vi "Initialize FGEN.vi"(8 "error in (no error)":errorcluster, 10 "FGEN Settings":T2, 11 "measurement context in":refnum<class "Measure Call Context.lvclass">) -> (0 "error out":errorcluster, 1 "Total Wfm Duration (s)":dbl, 2 "FGEN Sessions":T1, 3 "measurement context out":refnum<class "Measure Call Context.lvclass">)   [LabVIEW 2025, in "FGEN Arb Sequence Mode.lvclass"]
uses:
  FGEN Arb Sequence Mode.lvclass
  <vilib>/Plug-In SDKs/Measurements/Measure Call Context/Measure Call Context.lvclass
  <vilib>/Plug-In SDKs/Clients/Session Management V1/Session Reservation/Session Reservation.lvclass
  <instrlib>/niFgen/niFgen.llb/niFgen Output Mode.ctl
  <instrlib>/niFgen/niFgen.llb/niFgen Trigger Mode.ctl
  <vilib>/Plug-In SDKs/Clients/Session Management V1/Session Reservation/Initialize and Close Session Behavior.ctl
  <vilib>/Plug-In SDKs/Measurements/Measure Call Context/Reserve Sessions - NPin.vi
  <vilib>/Plug-In SDKs/Sessions/niFGEN/Initialize Sessions - 1Sess.vi
  <instrlib>/niFgen/niFgen.llb/niFgen Disable Start Trigger.vi
  <instrlib>/niFgen/niFgen.llb/niFgen Create Waveform (DBL).vi
  FGEN Arb Sequence Mode.lvclass/FGEN Arb Sequence Mode.ctl
  <vilib>/Plug-In SDKs/Sessions/niFGEN/NI Session Management niFGEN.lvlib
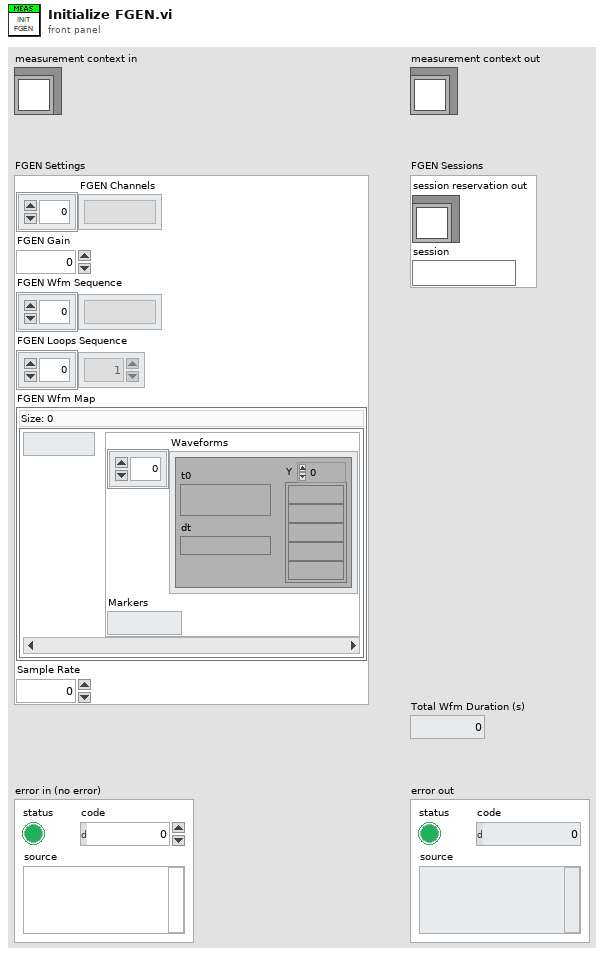
[diagram p1: front panel]
types:
  T1 = cluster{"session reservation out":refnum<class "Session Reservation.lvclass">, "session":refnum<k15>}
  T2 = cluster{"FGEN Channels":string[], "FGEN Gain":dbl, "FGEN Wfm Sequence":string[], "FGEN Loops Sequence":u32[], "FGEN Wfm Map":map{string, cluster{"Waveforms":waveform(dbl)[], "Markers":dbl}}, "Sample Rate":dbl}
  T3 = typedef "NI Session Management V1 Client.lvlib/Session Reservation.lvclass/Initialize and Close Session Behavior.ctl" = enum16{"Auto", "Initialize and Close", "Attach and Detach", "Initialize and Detach", "Attach and Close"}
  T4 = cluster{"Markers":i32, "Waveform Handle":i32, "Wfm Duration":dbl}
  T5 = map{string, cluster{"Markers":i32, "Waveform Handle":i32, "Wfm Duration":dbl}}
  T6 = typedef "niFgen Trigger Mode.ctl" = i32
  T7 = typedef "niFgen Output Mode.ctl" = u32
  T8 = map{string, cluster{"Waveforms":waveform(dbl)[], "Markers":dbl}}
  T9 = cluster{"Waveforms":waveform(dbl)[], "Markers":dbl}
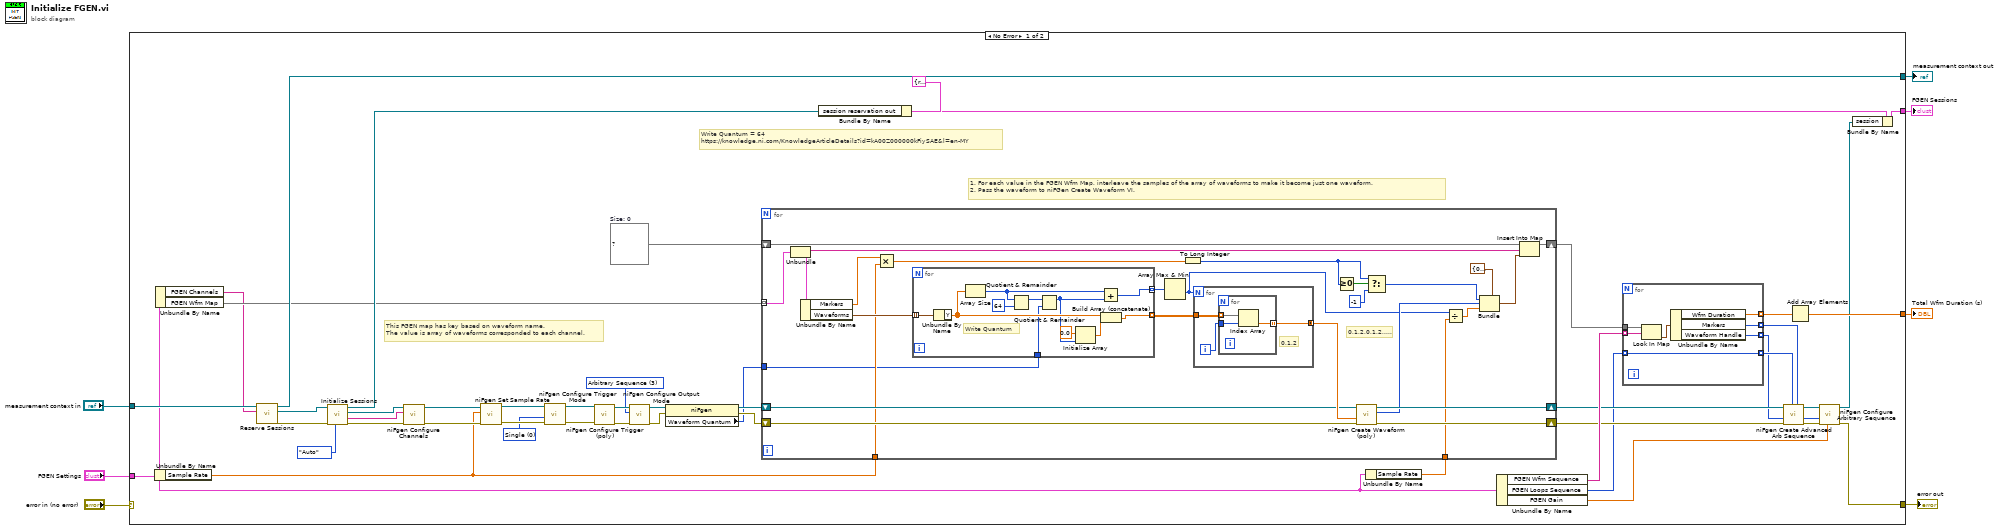
[diagram p0: block diagram]
diagram:
  n1 = case shown="No Error" "error in (no error)" {
    selector: "error in (no error)" -> [_ w109]
    tunnel: [w47 w109] -> w7
    tunnel: "FGEN Settings" -> [w22 _]
    tunnel: [w25 _] -> w4
    tunnel: "measurement context in" -> [w45 w108]
    tunnel: [w20 _] -> w2
    tunnel: [w39 w108] -> w1
    frame No Error {
      w36 = T5 {}  # Size: 0
      w46 = T6 0 items=["Single", "Continuous", "Stepped", "Burst"] ("Trigger Mode (default: 1=continuous)")
      w50 = T7 3 items=["Standard Function", "Frequency List", "Arbitrary Waveform", "Arbitrary Sequence", "Script"] ("Output Mode")
      # "Write Quantum = 64\nhttps://knowledge.ni.com/KnowledgeArticleDetails?id=kA00Z000000kFiySAE&l=en-MY"
      # "1. For each value in the FGEN Wfm Map, interleave the samples of the array of waveforms to make it become just one waveform.\n2. Pass the waveform to niFGen Create Waveform VI."
      # "This FGEN map has key based on waveform name. \nThe value is array of waveforms corresponded to each channel."
      n2 = Unbundle By Name(w22) -> ("Sample Rate"=w13:dbl)
      n3 = Unbundle By Name(w22) -> ("FGEN Channels"=w15:string[], "FGEN Wfm Map"=w34:T8)
      n4 = call-poly <vilib>:"Reserve Sessions.vi"("pin or relay names"=w15, "measurement context in"=w45) -> ("error out"=w43:errorcluster, "session reservation out"=w44:refnum<class "Session Reservation.lvclass">, "measurement context out"=w39:refnum<class "Measure Call Context.lvclass">)  [unwired: 7 in]
      n5 = call-poly <vilib>:"Initialize Sessions.vi"("initialize and close session behavior"=Initialize_and_Close_Session_Behavior."Auto", "error in"=w43, "session reservation in"=w44) -> ("error out"=w42:errorcluster, "channel list"=w14:string, "session"=w17:refnum<k15>, "session reservation out"=w37:refnum<class "Session Reservation.lvclass">)  [unwired: 5 in]
      n6 = call <instrlib>:"niFgen Configure Channels.vi"("error in (no error)"=w42, "Channels"=w14, "Instrument Handle"=w17) -> ("error out"=w18:errorcluster, "Instrument Handle Out"=w16:refnum<k15>)  [unwired: 7 in]
      n7 = call <instrlib>:"niFgen Set Sample Rate.vi"("error in (no error)"=w18, "Sample Rate (Samp/s)"=w13, "Instrument Handle"=w16) -> ("error out"=w55:errorcluster, "Instrument Handle Out"=w56:refnum<k15>)  [unwired: 7 in]
      n8 = call <instrlib>:"niFgen Configure Trigger Mode.vi"("error in (no error)"=w55, "Trigger Mode (default: 1=continuous)"=w46, "Instrument Handle"=w56) -> ("error out"=w53:errorcluster, "Instrument Handle Out"=w54:refnum<k15>)  [unwired: 7 in]
      n9 = call-poly <instrlib>:"niFgen Configure Trigger (poly).vi"("error in (no error)"=w53, "Instrument Handle"=w54) -> ("error out"=w51:errorcluster, "Instrument Handle Out"=w52:refnum<k15>)  [unwired: 8 in]
      n10 = call <instrlib>:"niFgen Configure Output Mode.vi"("error in (no error)"=w51, "Output Mode (default: 0=Standard Function)"=w50, "Instrument Handle"=w52) -> ("error out"=w35:errorcluster, "Instrument Handle Out"=w11:refnum<k15>)  [unwired: 6 in]
      n11 = property class="niFgen"(reference=w11, error in=w35) -> (reference out=w10:refnum<k15>, error out=w12:errorcluster, "Waveform Quantum"=w9:i32)
      n12 = Bundle By Name(cluster=T1 {"session reservation out"=refnum, "session"=""} ("FGEN Sessions"), "session reservation out"=w37) -> (w40:T1)
      n13 = Unbundle By Name(w22) -> ("Sample Rate"=w21:dbl)
      n14 = for {
        tunnel: w34 -> [w82] mode=indexing
        shift-right: [w83] -> w29
        shift-left: w10 -> [w86]
        shift-right: [w84] -> w28
        shift-left: w12 -> [w85]
        shift-right: [w71] -> w27
        shift-left: w36 -> [w72]
        tunnel: w21 -> [w74]
        tunnel: w13 -> [w69]
        tunnel: w9 -> [w64]
        # "0,1,2,0,1,2,...."
        n15 = Unbundle(w82) -> (w80:string, "output cluster"=w81:T9)
        n16 = Unbundle By Name(w81) -> ("Markers"=w78:dbl, "Waveforms"=w90:waveform(dbl)[])
        n17 = Multiply(x=w78, y=w69) -> (x*y=w70:dbl)
        n18 = for {
          tunnel: w90 -> [w107] mode=indexing
          tunnel: [w101] -> w88 mode=indexing
          tunnel: [w97] -> w89 mode=indexing
          tunnel: w64 -> [w103]
          # "Write Quantum"
          n19 = Unbundle By Name(w107) -> ("Y"=w106:dbl[])
          n20 = Array Size(array=w106) -> (size(s)=w99:i32)
          n21 = Quotient & Remainder(x=w99, y=64) -> (x-y*floor(x/y)=w104:i32)  [unwired: 1 out]
          n22 = Quotient & Remainder(x=w104, y=w103) -> (x-y*floor(x/y)=w98:i32)  [unwired: 1 out]
          n23 = Initialize Array(0.0 ("element"), w98) -> (w100:dbl[])
          n24 = Add(x=w99, y=w98) -> (x+y=w97:i32)
          n25 = Build Array (concatenate)(w106, w100) -> (w101:dbl[])
        }
        n26 = Array Max & Min(array=w89) -> (min value=w75:i32)  [unwired: 3 out]
        n27 = To Long Integer(number=w70) -> (32bit integer=w66:i32)
        n28 = for {
          N: w75 -> [_]
          tunnel: w88 -> [w93]
          tunnel: [w91] -> w87 mode=concatenating
          i -> [w92]
          # "0,1,2"
          n29 = for {
            tunnel: w93 -> [w96] mode=indexing
            tunnel: w92 -> [w95]
            tunnel: [w94] -> w91 mode=indexing
            n30 = Index Array(array=w96, index=w95) -> (element=w94:dbl)
          }
        }
        n31 = Greater Or Equal To 0?(x=w66) -> (x >= 0?=w67:bool)
        n32 = call-poly <instrlib>:"niFgen Create Waveform (poly).vi"("error in (no error)"=w85, "Waveform Data Array"=w87, "Instrument Handle"=w86) -> ("error out"=w84:errorcluster, "Waveform Handle"=w77:i32, "Instrument Handle Out"=w83:refnum<k15>)  [unwired: 6 in]
        n33 = Select(t=w66, s=w67, f=-1) -> (s? t:f=w68:i32)
        n34 = Divide(x=w75, y=w74) -> (x/y=w73:dbl)
        n35 = Bundle(cluster=T4 {"Markers"=0, "Waveform Handle"=0, "Wfm Duration"=0.0} ("value"), "Markers"=w68, "Waveform Handle"=w77, "Wfm Duration"=w73) -> (w76:T4)
        n36 = Insert Into Map(map in=w72, key=w80, value=w76) -> (map out=w71:T5)  [unwired: 2 out]
      }
      n37 = Unbundle By Name(w22) -> ("FGEN Wfm Sequence"=w49:string[], "FGEN Loops Sequence"=w8:u32[], "FGEN Gain"=w48:dbl)
      n38 = for {
        tunnel: w49 -> [w63] mode=indexing
        tunnel: [w62] -> w23 mode=indexing
        tunnel: [w61] -> w24 mode=indexing
        tunnel: [w57] -> w33 mode=indexing
        tunnel: w27 -> [w60]
        tunnel: [w58] -> w26 mode=indexing
        tunnel: w8 -> [w57] mode=indexing
        n39 = Look In Map(map=w60, key=w63) -> (value=w59:T4)  [unwired: 1 in, 1 out]
        n40 = Unbundle By Name(w59) -> ("Wfm Duration"=w58:dbl, "Markers"=w61:i32, "Waveform Handle"=w62:i32)
      }
      n41 = call <instrlib>:"niFgen Create Advanced Arb Sequence.vi"("Marker Location Array"=w24, "Loop Counts Array"=w33, "error in (no error)"=w28, "Waveform Handles Array"=w23, "Instrument Handle"=w29) -> ("error out"=w32:errorcluster, "Sequence Handle"=w30:i32, "Instrument Handle Out"=w31:refnum<k15>)  [unwired: 3 in, 1 out]
      n42 = Add Array Elements(numeric array=w26) -> (sum=w25:dbl)
      n43 = call <instrlib>:"niFgen Configure Arbitrary Sequence.vi"("Gain"=w48, "error in (no error)"=w32, "Sequence Handle"=w30, "Instrument Handle"=w31) -> ("error out"=w47:errorcluster, "Instrument Handle Out"=w19:refnum<k15>)  [unwired: 6 in]
      n44 = Bundle By Name(cluster=w40, "session"=w19) -> (w20:T1)
    }
    frame Error {
    }
  }
  "error out" <- w7
  "Total Wfm Duration (s)" <- w4
  "FGEN Sessions" <- w2
  "measurement context out" <- w1
